vi "PromTest2 - Get Metrics.vi"(7 "LabVIEW Web Service Request":refnum<class "Web Request.lvclass">, 11 "Registry":string="_default_registry") -> ()   [LabVIEW 2020]
uses:
  <vilib>/wsapi/Web Request.lvclass
  src/metrics/metric/Metric.lvclass
  src/registry/session/Registry Session.lvclass
  <vilib>/Utility/error.llb/DialogType.ctl
panel:
  # "Use the Web Service Request input terminal to call the VIs on the Web Services palette. Do not remove it from the connector pane unless you don't need access to the palette."
  # "Each additional control wired to the connector pane will be available as an input in the URL. To include an indicator in terminal-mode output (the default setting), it must also be wired to the connector pane."
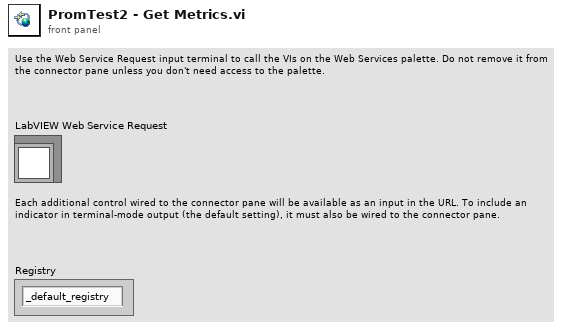
[diagram p1: front panel]
types:
  T1 = typedef "Registry.lvlib/Registry Session.lvclass/Session Handle.ctl" = refnum<data-value>
  T2 = typedef "DialogType.ctl" = u16
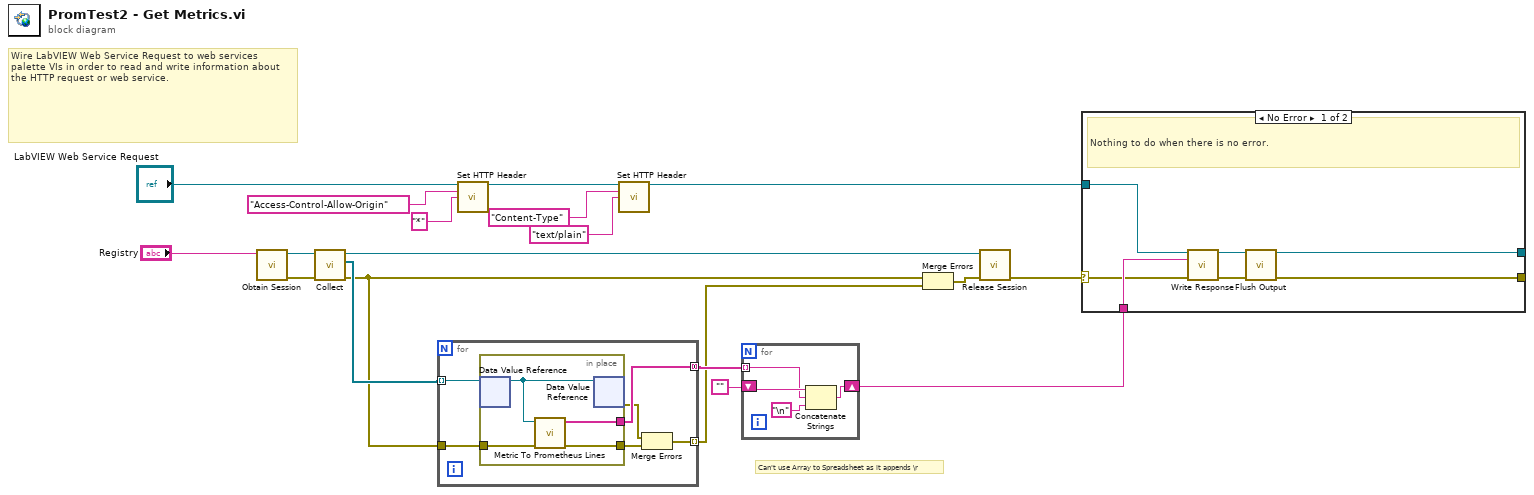
[diagram p0: block diagram]
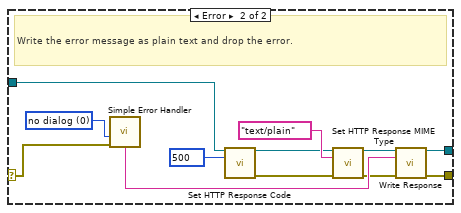
[diagram p2: hidden frame]
diagram:
  # "Can't use Array to Spreadsheet as it appends \\r"
  # "Wire LabVIEW Web Service Request to web services palette VIs in order to read and write information about the HTTP request or web service."
  n1 = call "Obtain Session.vi"("Session  Name ()"="Registry") -> ("error out"=w14:errorcluster, "Session Handle"=w15:T1)  [unwired: 9 in]
  n2 = call "Collect.vi"("error in (no error)"=w14, "Session Handle in"=w15) -> ("error out"=w2:errorcluster, "Metrics"=w7:refnum<data-value>[], "Session Handle out"=w13:T1)  [unwired: 7 in]
  n3 = for {
    tunnel: w7 -> [w25] mode=indexing
    tunnel: [w24] -> w6 mode=concatenating
    tunnel: w2 -> [w21]
    tunnel: [w20] -> w1 mode=indexing
    n4 = in-place {
      in-place-border: [w28] -> w24
      in-place-border: [w27] -> w22
      in-place-border: w21 -> [w26]
      n5 = in-place-dvr #1(w25) -> (w29:refnum<class "Metric.lvclass">)  [unwired: 1 out]
      n6 = call-dynamic "Metric To Prometheus Lines.vi"("error in (no error)"=w26, "Metrics.lvlib:Metric.lvclass"=w29) -> ("error out"=w27:errorcluster, "Prometheus Lines"=w28:string[])  [unwired: 8 in]
      n7 = in-place-dvr #1(w29) -> (w23:errorcluster)  [unwired: 1 out]
    }
    n8 = Merge Errors(w23, w22) -> (w20:errorcluster)
  }
  n9 = call <vilib>:"Set HTTP Header.vi"("LabVIEW Web Service Request"="LabVIEW Web Service Request", "header"="Access-Control-Allow-Origin", "header value"="*") -> ("LabVIEW Web Service Request out"=w10:refnum<class "Web Request.lvclass">)  [unwired: 11 in, 1 out]
  n10 = call <vilib>:"Set HTTP Header.vi"("LabVIEW Web Service Request"=w10, "header"="Content-Type", "header value"="text/plain") -> ("LabVIEW Web Service Request out"=w5:refnum<class "Web Request.lvclass">)  [unwired: 11 in, 1 out]
  n11 = for {
    tunnel: w6 -> [w31] mode=indexing
    shift-right: [w30] -> w3
    shift-left: "" -> [w33]
    n12 = Concatenate Strings(w33, w31, "\n") -> (w30:string)
  }
  n13 = Merge Errors(w2, w1) -> (w9:errorcluster)
  n14 = call "Release Session.vi"("error in (no error)"=w9, "Session Handle"=w13) -> ("error out"=w4:errorcluster)  [unwired: 9 in]
  n15 = case shown="No Error" w4 {
    selector: w4 -> [w35 w48]
    tunnel: w5 -> [w39 w43]
    tunnel: [w38 w50] -> _
    tunnel: [w34 w49] -> _
    tunnel: w3 -> [w37 _]
    frame No Error {
      # "Nothing to do when there is no error."
      n16 = call <vilib>:"Write Response.vi"("LabVIEW Web Service Request"=w39, "response string"=w37, "error in (no error)"=w35) -> ("LabVIEW Web Service Request out"=w40:refnum<class "Web Request.lvclass">, "error out"=w36:errorcluster)  [unwired: 11 in]
      n17 = call <vilib>:"Flush Output.vi"("LabVIEW Web Service Request"=w40, "error in (no error)"=w36) -> ("LabVIEW Web Service Request out"=w38:refnum<class "Web Request.lvclass">, "error out"=w34:errorcluster)  [unwired: 12 in]
    }
    frame Error {
      w44 = 500 items=["100"=100, "101"=101, "200"=200, "201"=201, "202"=202, "203"=203, "204"=204, "205"=205, "206"=206, "300"=300, "301"=301, "302"=302, "303"=303, "304"=304, "305"=305, "306"=306, "307"=307, "400"=400, "401"=401, "402"=402, "403"=403, "404"=404, "405"=405, "406"=406, "407"=407, "408"=408, "409"=409, "410"=410, "411"=411, "412"=412, "413"=413, "414"=414, "415"=415, "416"=416, "417"=417, "500"=500, "501"=501, "502"=502, "503"=503, "504"=504, "505"=505] ("response code (200)")
      w51 = T2 0 items=["no dialog", "OK message", "continue or stop message", "OK message + warnings", "continue/stop + warnings"] ("type of dialog (OK msg:1)")
      # "Write the error message as plain text and drop the error."
      n18 = call <vilib>:"Simple Error Handler.vi"("type of dialog (OK msg:1)"=w51, "error in (no error)"=w48) -> ("message"=w52:string)  [unwired: 3 in, 4 out]
      n19 = call <vilib>:"Set HTTP Response Code.vi"("LabVIEW Web Service Request"=w43, "response code (200)"=w44) -> ("LabVIEW Web Service Request out"=w42:refnum<class "Web Request.lvclass">, "error out"=w45:errorcluster)  [unwired: 12 in]
      n20 = call <vilib>:"Set HTTP Response MIME Type.vi"("LabVIEW Web Service Request"=w42, "MIME type (text/html)"="text/plain", "error in (no error)"=w45) -> ("LabVIEW Web Service Request out"=w41:refnum<class "Web Request.lvclass">, "error out"=w47:errorcluster)  [unwired: 11 in]
      n21 = call <vilib>:"Write Response.vi"("LabVIEW Web Service Request"=w41, "response string"=w52, "error in (no error)"=w47) -> ("LabVIEW Web Service Request out"=w50:refnum<class "Web Request.lvclass">, "error out"=w49:errorcluster)  [unwired: 11 in]
    }
  }
